vi "拉取dll.vi"(10 "名称或相对路径":string="FreeMem.zip", 11 "服务器":T1={"host"="27.154.58.30", "port"=8020, "user"="std", "password"="std23506", "远端地址"="/微站/四代/一体化微型水质监测站.exe"}) -> (0 "error out":errorcluster caption="错误输出")   [LabVIEW 2016, in "数据传输系统-04.lvlib" / "update.lvlib"]
uses:
  update.lvlib
  <vilib>/httpClient/POSTBuffer.vi
  <vilib>/httpClient/LabVIEWHTTPClient.lvlib
panel:
  out "headers":string caption="头部"
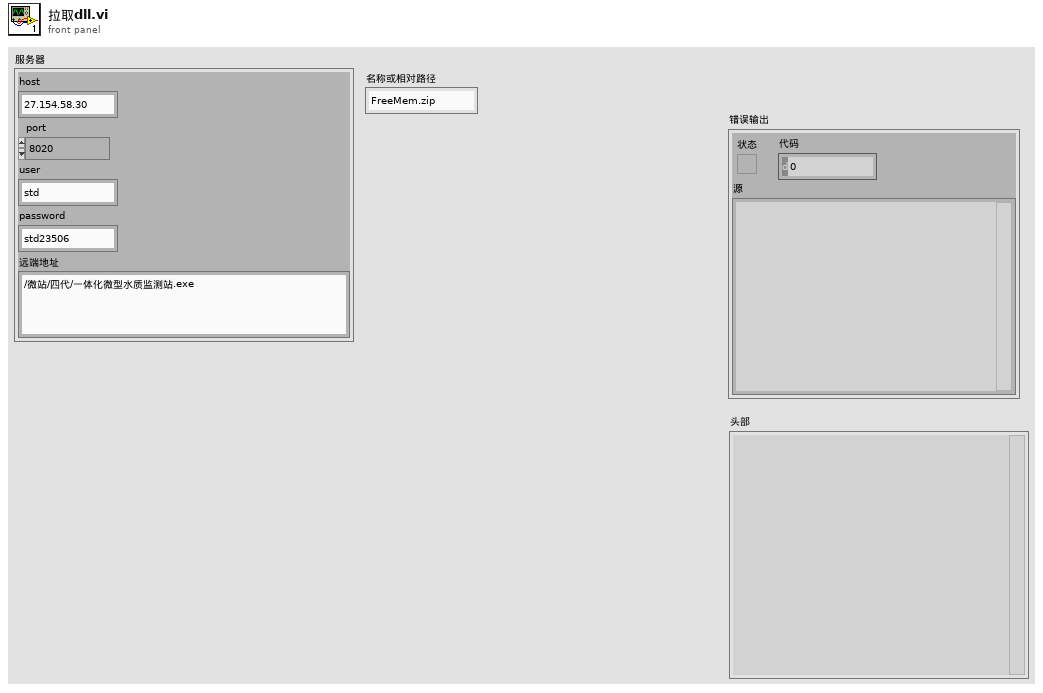
[diagram p1: front panel]
types:
  T1 = cluster{"host":string, "port":u16, "user":string, "password":string, "远端地址":string}
  T2 = typedef "LabVIEWHTTPClient.lvlib/ClientHandle.ctl" = refnum<k1>
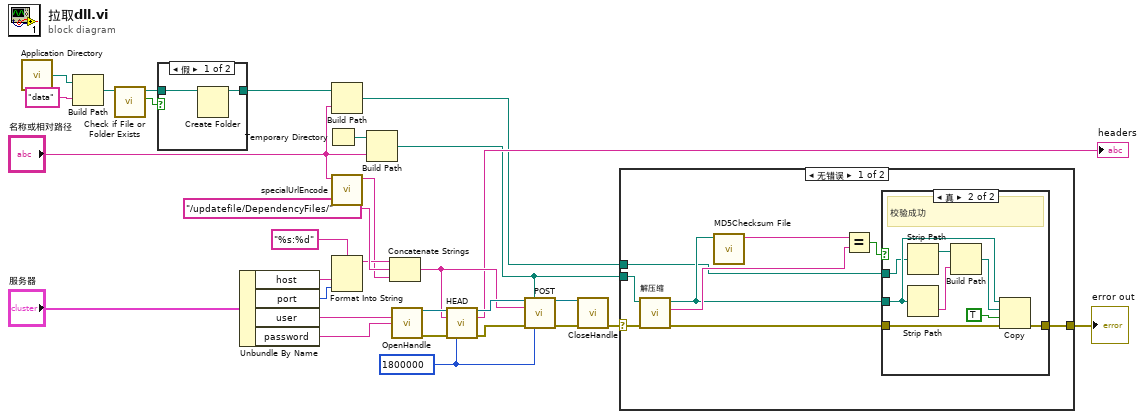
[diagram p0: block diagram]
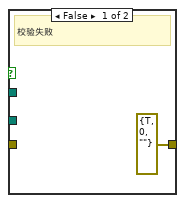
[diagram p2: hidden frame]
diagram:
  w17 = 1800000 ("timeout (10000)")
  n1 = call <vilib>:"Application Directory.vi"() -> ("Application Directory"=w10:path)
  n2 = Build Path(base path=w10, name or relative path="data" ("名称或相对路径")) -> (appended path=w11:path)
  n3 = call <vilib>:"Check if File or Folder Exists.vi"("path"=w11) -> ("file or folder exists?"=w12:bool, "dup path"=w13:path)  [unwired: 8 in, 1 out]
  n4 = case shown="假" w12 {
    tunnel: w13 -> [w32 w33]
    tunnel: [w31 w33] -> w8
    frame False {
      n5 = Create Folder(path (use dialog)=w32) -> (created path=w31:path)  [unwired: 2 in, 2 out]
    }
    frame True {
    }
  }
  n6 = Unbundle By Name("服务器") -> ("host"=w28:string, "port"=w27:u16, "user"=w16:string, "password"=w15:string)
  n7 = Temporary Directory() -> (w3:path)
  n8 = Build Path(base path=w8, name or relative path="名称或相对路径") -> (appended path=w4:path)
  n9 = call "specialUrlEncode.vi"("str"="名称或相对路径") -> ("UrlEncode"=w24:string)  [unwired: 10 in]
  n10 = Format Into String(format string="%s:%d" ("格式字符串"), w28, w27) -> (resulting string=w25:string)  [unwired: 2 in, 1 out]
  n11 = Build Path(base path=w3, name or relative path="名称或相对路径") -> (appended path=w2:path)
  n12 = Concatenate Strings(w25, "/updatefile/DependencyFiles/", w24) -> (w14:string)
  n13 = call <vilib>:"OpenHandle.vi"("username"=w16, "password"=w15) -> ("client handle out"=w21:T2, "error out"=w19:errorcluster)  [unwired: 12 in]
  n14 = call <vilib>:"HEAD.vi"("client handle"=w21, "url"=w14, "error in (no error)"=w19, "timeout (10000)"=w17) -> ("client handle out"=w20:T2, "headers"=→"headers":string, "error out"=w18:errorcluster)  [unwired: 9 in]
  n15 = call-poly <vilib>:"POST.vi"("client handle"=w20, "output file"=w2, "url"=w14, "error in (no error)"=w18, "timeout (10000)"=w17) -> ("client handle out"=w23:T2, "error out"=w22:errorcluster)  [unwired: 7 in, 2 out]
  n16 = call <vilib>:"CloseHandle.vi"("client handle"=w23, "error in (no error)"=w22) -> ("error out"=w7:errorcluster)  [unwired: 13 in]
  n17 = case shown="无错误" w7 {
    selector: w7 -> [w39 w52]
    tunnel: w2 -> [w35 _]
    tunnel: [w41 w52] -> w6
    tunnel: w4 -> [w34 _]
    frame No Error {
      n18 = call "解压缩.vi"("error in (no error)"=w39, "Zip file"=w35) -> ("error out"=w38:errorcluster, "MD5"=w40:string, "待校验的文件路径"=w36:path)  [unwired: 7 in]
      n19 = call <vilib>:"MD5Checksum File.vi"("Path"=w36) -> ("MD5 message-digest"=w42:string)  [unwired: 9 in, 1 out]
      n20 = Equal?(x=w42, y=w40) -> (x = y?=w37:bool)
      n21 = case shown="真" w37 {
        tunnel: w38 -> [_ w45]
        tunnel: [errorcluster {"status"=TRUE, "code"=0, "source"=""} ("error IO") w44] -> w41
        tunnel: w36 -> [_ w50]
        tunnel: w34 -> [_ w49]
        frame False {
          # "校验失败"
        }
        frame True {
          # "校验成功"
          n22 = Strip Path(path=w49) -> (stripped path=w48:path)  [unwired: 1 out]
          n23 = Strip Path(path=w50) -> (name=w47:string)  [unwired: 1 out]
          n24 = Build Path(base path=w48, name or relative path=w47) -> (appended path=w46:path)
          n25 = Copy(8:w45, 9:TRUE ("覆盖(F)"), 10:w46, 11:w50) -> (0:w44:errorcluster)  [unwired: 1 in, 2 out]
        }
      }
    }
    frame Error {
    }
  }
  "error out" <- w6
